vi "getPulseDuration.vi"(10 "target microL/pulse":dbl format="%#_13g", 11 "Probe #":u8) -> (3 "Pulse Duration":dbl)   [LabVIEW 2014]
uses:
  <vilib>/Analysis/6fits.llb/Curve Fitting Criteria.ctl
  <vilib>/Utility/file.llb/Read From Spreadsheet File (string).vi
  <vilib>/regexp/Match Regular Expression.xnode
  <vilib>/Analysis/NI_AALPro.lvlib
panel:
  out "string":string[](array[string])
  out "substring":string
  out "Numeric":i32
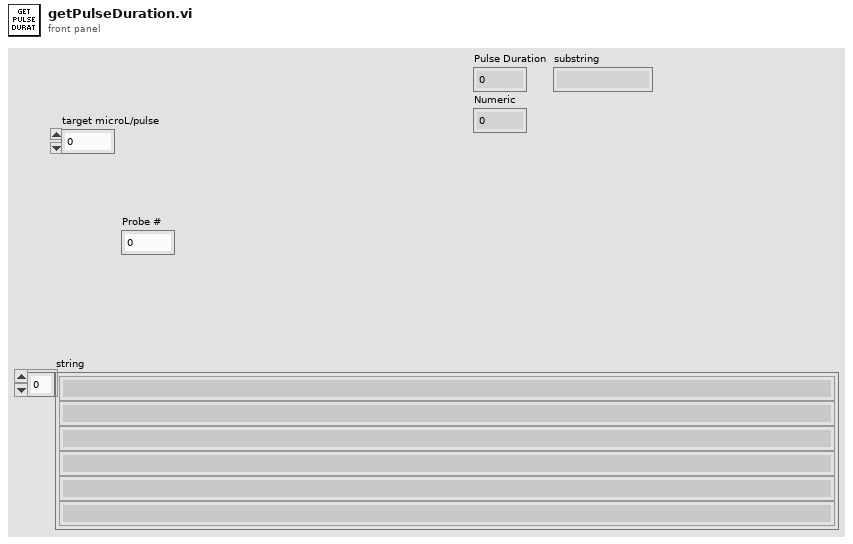
[diagram p1: front panel]
types:
  T1 = typedef "NI_AALPro.lvlib/Curve Fitting Criteria.ctl" = u16
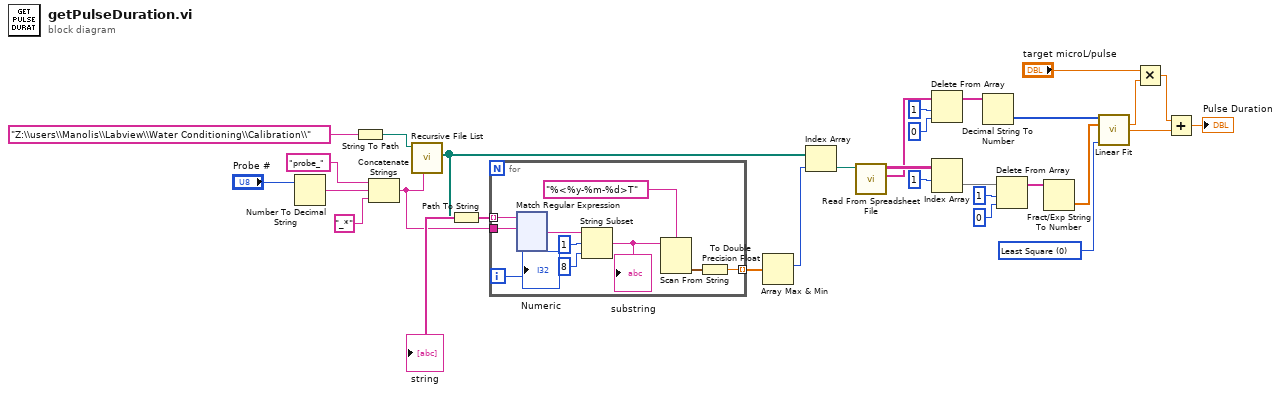
[diagram p0: block diagram]
diagram:
  w15 = T1 0 items=["Least Square", "Least Absolute Residual", "Bisquare"] ("method")
  n1 = Number To Decimal String(number="Probe #") -> (decimal integer string=w29:string)  [unwired: 1 in]
  n2 = String To Path(string="Z:\\users\\Manolis\\Labview\\Water Conditioning\\Calibration\\") -> (path=w26:path)
  n3 = Concatenate Strings("probe_", w29, "_*" ("string")) -> (w23:string)
  n4 = call <vilib>:"Recursive File List.vi"("pattern"=w23, "Folder Path"=w26) -> ("All Files in Dir"=w21:path[])  [unwired: 5 in, 4 out]
  n5 = Path To String(path=w21) -> (string=w24:string[])
  "string" <- w24
  n6 = for {
    tunnel: w24 -> [w40] mode=indexing
    tunnel: w23 -> [w39]
    tunnel: [w32] -> w22 mode=indexing
    i -> [w31]
    n7 = xnode "Match Regular Expression"("input string"=w40, "regular expression"=w39) -> ("after match"=w38:string)  [unwired: 4 in, 4 out]
    n8 = String Subset(string=w38, offset (0)=1, length (rest)=8 ("length (rest)")) -> (substring=w34:string)
    "substring" <- w34
    n9 = Scan From String(format string="%<%y-%m-%d>T", input string=w34) -> (output 1=w33:timestamp)  [unwired: 3 in, 3 out]
    n10 = To Double Precision Float(number=w33) -> (double precision float=w32:dbl)
    "Numeric" <- w31
  }
  n11 = Array Max & Min(array=w22) -> (max index (indices)=w20:i32)  [unwired: 3 out]
  n12 = Index Array(array=w21, index=w20) -> (element=w13:path)
  n13 = call-poly <vilib>:"Read From Spreadsheet File.vi"("file path (dialog if empty)"=w13) -> ("first row"=w2:string[], "all rows"=w11:string[][])  [unwired: 6 in, 3 out]
  n14 = Delete From Array(array=w2, length=1, index=0) -> (array with subset deleted=w1:string[])  [unwired: 1 out]
  n15 = Index Array(array=w11, index (row)=1) -> (element=w8:string[])  [unwired: 1 in]
  n16 = Decimal String To Number(string=w1) -> (number=w12:i32[])  [unwired: 2 in, 1 out]
  n17 = Delete From Array(array=w8, length=1, index=0) -> (array with subset deleted=w5:string[])  [unwired: 1 out]
  n18 = Fract/Exp String To Number(string=w5) -> (number=w9:dbl[])  [unwired: 3 in, 1 out]
  n19 = call <vilib>:"Linear Fit.vi"("Y"=w12, "X"=w9, "method"=w15) -> ("slope"=w19:dbl, "intercept"=w17:dbl)  [unwired: 8 in, 3 out]
  n20 = Multiply(x="target microL/pulse", y=w19) -> (x*y=w18:dbl)
  n21 = Add(x=w18, y=w17) -> (x+y=→"Pulse Duration":dbl)
